vi "Hardware - VRHall-1 Host.vi"() -> ()   [LabVIEW 2015, in "ECS-Host.lvlib"]
uses:
  ECS-Host.lvlib
panel:
  in  "SignalConfig":u32
  in  "_Signal Config":bool[](array[boolean])=[FALSE, FALSE, FALSE, FALSE, FALSE, FALSE, FALSE, FALSE, FALSE, FALSE, FALSE, FALSE, FALSE, FALSE, FALSE, FALSE, FALSE, FALSE, FALSE, FALSE, FALSE, FALSE, FALSE, FALSE, FALSE, FALSE, FALSE, FALSE, FALSE, FALSE, FALSE, FALSE]
  out "_Channel Names":string[](array[string])
  out "Freq":sgl[](array[numeric]) format="%#_5f"
  out "DC":sgl[](array[numeric]) step=0.1 format="%.2f"
  out "PulseWidth":sgl[](array[numeric]) step=0.1 format="%#_5f"
  in  "_Digital_InvertConfig_Array":bool[](array[boolean])=[FALSE, FALSE, FALSE, FALSE, FALSE, FALSE, FALSE, FALSE, FALSE, FALSE, FALSE, FALSE, FALSE, FALSE, FALSE, FALSE, FALSE, FALSE, FALSE, FALSE, FALSE, FALSE, FALSE, FALSE, FALSE, FALSE, FALSE, FALSE, FALSE, FALSE, FALSE, FALSE]
  in  "DigitalFilt":sgl[](array[numeric]) format="%#.2f"
  out "_VRHall_DigInput_Array":bool[](array[boolean])
  out "FPGAWriteError":bool
  out "FPGAReadError":bool
  in  "DigitalInvertConfig":u32
  out "DigitalInputBooleanArray":u32
  # "Channel Name"
  # "State"
  # "Freq [Hz]"
  # "DC [%]"
  # "PW [ms] [msec]"
  # "Invert Input"
  # "Filter [us]"
  # "Config"
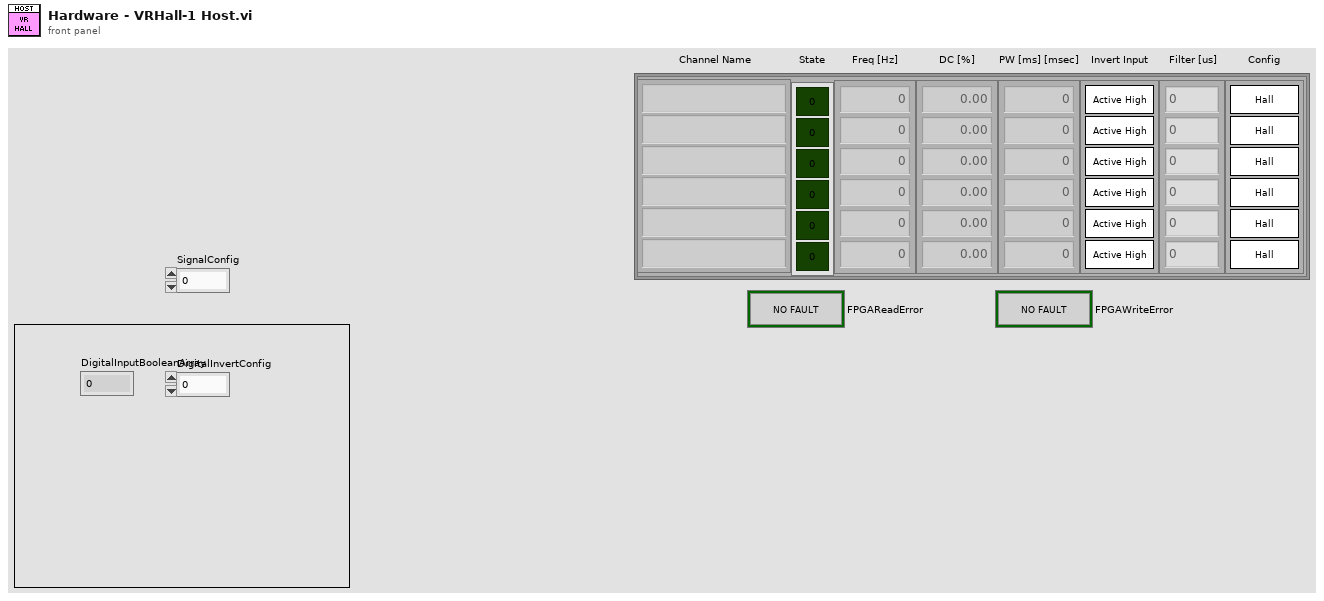
[diagram p1: front panel]
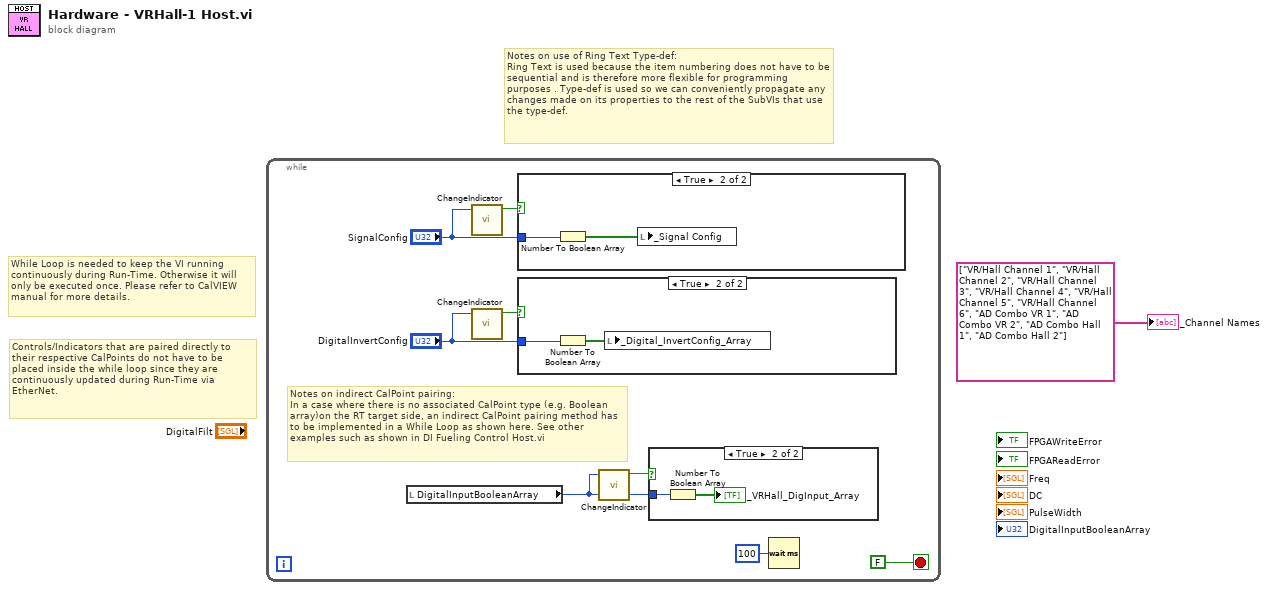
[diagram p0: block diagram]
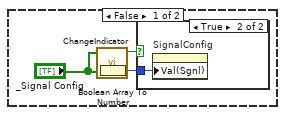
[diagram p2: hidden frame]
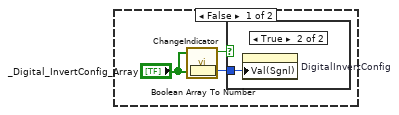
[diagram p4: hidden frame]
diagram:
  # "Notes on use of Ring Text Type-def:\nRing Text is used because the item numbering does not have to be sequential and is therefore more flexible for programming purposes . Type-def is used so we can conveniently propagate any changes made on its properties to the rest of the SubVIs that use the type-def."
  # "While Loop is needed to keep the VI running\ncontinuously during Run-Time. Otherwise it will only be executed once. Please refer to CalVIEW manual for more details."
  # "Controls/Indicators that are paired directly to their respective CalPoints do not have to be placed inside the while loop since they are continuously updated during Run-Time via EtherNet."
  n1 = while {
    stop <- FALSE stop-if-true
    # "Notes on indirect CalPoint pairing:\nIn a case where there is no associated CalPoint type (e.g. Boolean array)on the RT target side, an indirect CalPoint pairing method has to be implemented in a While Loop as shown here. See other examples such as shown in DI Fueling Control Host.vi"
    n2 = local read "DigitalInputBooleanArray"() -> (w7:u32)
    n3 = call "ChangeIndicator.vi"("Input"="SignalConfig") -> ("Change"=w2:bool)  [unwired: 9 in]
    n4 = call "ChangeIndicator.vi"("Input"="DigitalInvertConfig") -> ("Change"=w5:bool)  [unwired: 9 in]
    n5 = case shown="True" w2 {
      tunnel: "SignalConfig" -> [_ w15]
      frame False {
        n6 = call "ChangeIndicator.vi"("Input"="_Signal Config") -> ("Change"=w11:bool)  [unwired: 9 in]
        n7 = Boolean Array To Number(Boolean array="_Signal Config") -> (number=w12:u32)
        n8 = case shown="True" w11 {
          tunnel: w12 -> [_ w13]
          frame False {
          }
          frame True {
            n9 = property on="SignalConfig" class="DigNum (strict)"("Val(Sgnl)"=w13) -> ()  [unwired: 2 in, 2 out]
          }
        }
      }
      frame True {
        n10 = Number To Boolean Array(number=w15) -> (Boolean array=w14:bool[])
        n11 = local write "_Signal Config"(w14) -> ()
      }
    }
    n12 = case shown="True" w5 {
      tunnel: "DigitalInvertConfig" -> [_ w21]
      frame False {
        n13 = call "ChangeIndicator.vi"("Input"="_Digital_InvertConfig_Array") -> ("Change"=w17:bool)  [unwired: 9 in]
        n14 = Boolean Array To Number(Boolean array="_Digital_InvertConfig_Array") -> (number=w18:u32)
        n15 = case shown="True" w17 {
          tunnel: w18 -> [_ w19]
          frame False {
          }
          frame True {
            n16 = property on="DigitalInvertConfig" class="DigNum (strict)"("Val(Sgnl)"=w19) -> ()  [unwired: 2 in, 2 out]
          }
        }
      }
      frame True {
        n17 = Number To Boolean Array(number=w21) -> (Boolean array=w20:bool[])
        n18 = local write "_Digital_InvertConfig_Array"(w20) -> ()
      }
    }
    n19 = call "ChangeIndicator.vi"("Input"=w7) -> ("Change"=w6:bool)  [unwired: 9 in]
    n20 = case shown="True" w6 {
      tunnel: w7 -> [_ w22]
      frame False {
      }
      frame True {
        n21 = Number To Boolean Array(number=w22) -> (Boolean array=→"_VRHall_DigInput_Array":bool[])
      }
    }
    n22 = Wait (ms)(milliseconds to wait=u32 100) -> ()  [unwired: 1 out]
  }
  "_Channel Names" <- string[] ["VR/Hall Channel 1", "VR/Hall Channel 2", "VR/Hall Channel 3", "VR/Hall Channel 4", "VR/Hall Channel 5", "VR/Hall Channel 6", "AD Combo VR 1", "AD Combo VR 2", "AD Combo Hall 1", "AD Combo Hall 2"]
